vi "Write to Text Log File (U8).vi"(6 "Data":u8[][](array[numeric]), 8 "error in (no error)":errorcluster, 9 "Channel Names in":string[](array[string]), 10 "Group Names in":string[](array[string]), 11 "Text Log File in":refnum<class "Text Log File.lvclass">) -> (0 "error out":errorcluster, 3 "Text Log File out":refnum<class "Text Log File.lvclass">)   [LabVIEW 2015, in "Text Log File.lvclass"]
doc: "Writes data to the text file using the specified delimiter and format string. The channel and group names are ignored. The header for the file should be written in advance using Write Log Header.vi."
uses:
  Text Log File.lvclass
  Text Log File.lvclass/Text Log File.ctl
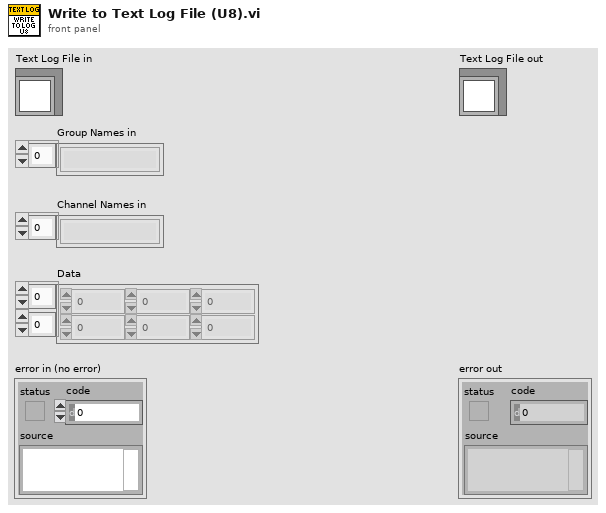
[diagram p1: front panel]
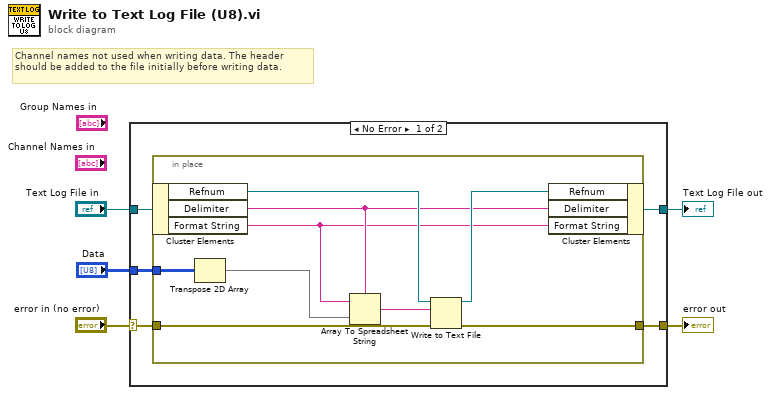
[diagram p0: block diagram]
diagram:
  # "Channel names not used when writing data. The header should be added to the file initially before writing data."
  n1 = case shown="No Error" "error in (no error)" {
    selector: "error in (no error)" -> [w6 w20]
    tunnel: [w10 w21] -> w5
    tunnel: "Data" -> [w9 _]
    tunnel: [w8 w20] -> w3
    tunnel: "Text Log File in" -> [w7 w21]
    frame No Error {
      n2 = in-place {
        in-place-border: w6 -> [w19]
        in-place-border: w9 -> [w18]
        in-place-border: [w16] -> w8
        n3 = in-place-cluster #1(w7) -> ("Refnum"=w15:refnum<file>, "Delimiter"=w13:string, "Format String"=w12:string)
        n4 = Transpose 2D Array(2D array=w18) -> (transposed array=w14:u8[][])
        n5 = Array To Spreadsheet String(delimiter (Tab)=w13, array=w14, 3:w12) -> (spreadsheet string=w11:string)
        n6 = Write to Text File(file (use dialog)=w15, text=w11, error in=w19) -> (refnum out=w17:refnum<file>, error out=w16:errorcluster)  [unwired: 1 in, 1 out]
        n7 = in-place-cluster #1("Refnum"=w17, "Delimiter"=w13, "Format String"=w12) -> (w10:refnum<class "Text Log File.lvclass">)
      }
    }
    frame Error {
    }
  }
  "error out" <- w3
  "Text Log File out" <- w5
